vi "DDS Write Register.vi"(6 "channel number (1)":u8=1 min=1 max=4 step=1, 8 "error in (no error)":errorcluster, 9 "Write Data":u8[](array[numeric]), 10 "Register":T3, 11 "DDS ref in":T1={"NI USB-8451 device reference"="", "DIO port"=0, "Serial Clock Rate [kHz]"=1000}) -> (0 "error out":errorcluster, 3 "DDS ref out":T1={"NI USB-8451 device reference"="", "DIO port"=0, "Serial Clock Rate [kHz]"=1000})   [LabVIEW 2013]
doc: "Writes data to the specified register in the specified channel. The number of bytes written must equal the register size."
uses:
  AD9910 registers.ctl
  DDS_box_device_reference.ctl
  <vilib>/ni845x/ni845x.llb/ni845xControl.ctl
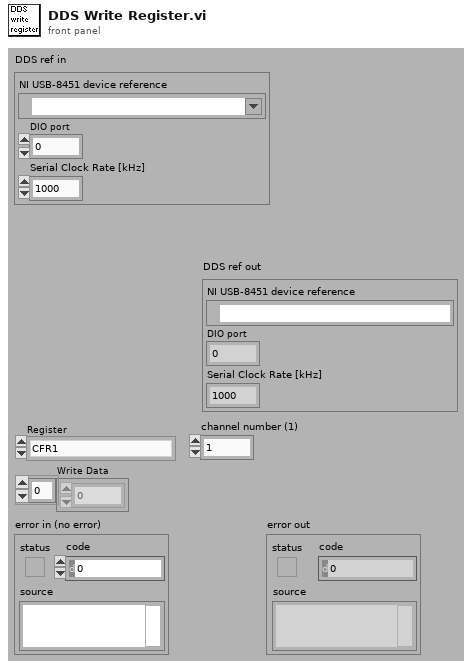
[diagram p1: front panel]
types:
  T1 = typedef "DDS_box_device_reference.ctl" = cluster{"NI USB-8451 device reference":T2, "DIO port":u8, "Serial Clock Rate [kHz]":u16}
  T2 = typedef "ni845xControl.ctl" = refnum<k21>
  T3 = typedef "AD9910 registers.ctl" = enum16{"CFR1", "CFR2", "CFR3", "Auxiliary DAC Control", "I/0 Update Rate", "Frequency Tuning Word", "Phase Offset Word", "Amplitude Scale Factor", "Multichip Sync", "Digital Ramp Limit", "Digital Ramp Step Size", "Digital Ramp Rate", "Single Tone Profile 0", "Single Tone Profile 1", "Single Tone Profile 2", "Single Tone Profile 3", "Single Tone Profile 4", "Single Tone Profile 5", "Single Tone Profile 6", "Single Tone Profile 7", "RAM Profile 0", "RAM Profile 1", "RAM Profile 2", "RAM Profile 3", "RAM Profile 4", "RAM Profile 5", "RAM Profile 6", "RAM Profile 7", "RAM"}
  T4 = typedef "ni845xSpiScriptControl.ctl" = refnum<k20>
  T5 = typedef "DDS CS pins.ctl" = enum8{"IO reset", "Ch. 4 CS", "Ch. 3 CS", "Ch. 2 CS", "Ch. 1 CS"}
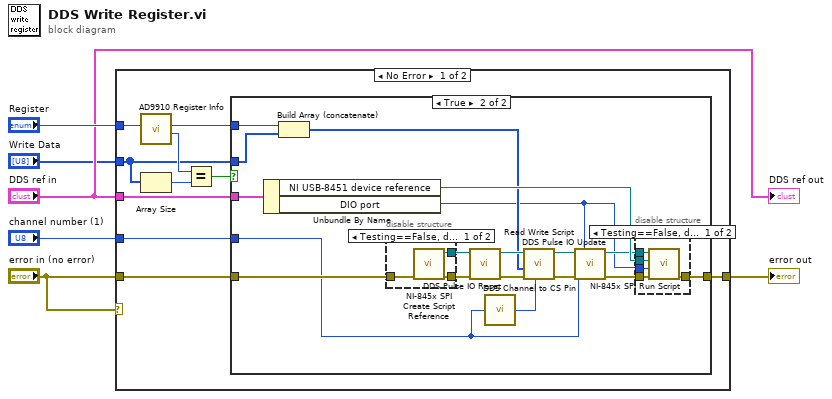
[diagram p0: block diagram]
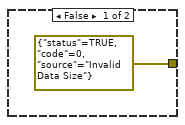
[diagram p2: hidden frame]
diagram:
  n1 = case shown="No Error" "error in (no error)" {
    tunnel: "error in (no error)" -> [w16 w46]
    tunnel: "DDS ref in" -> [w15 _]
    tunnel: "Register" -> [w14 _]
    tunnel: [w8 w46] -> w4
    tunnel: "Write Data" -> [w10 _]
    tunnel: "channel number (1)" -> [w7 _]
    frame No Error {
      n2 = call "AD9910 Register Info.vi"("Register"=w14) -> ("Number of Bytes"=w13:i32, "Address"=w9:u8)  [unwired: 9 in]
      n3 = Array Size(array=w10) -> (size(s)=w12:i32)
      n4 = Equal?(x=w13, y=w12) -> (x = y?=w11:bool)
      n5 = case shown="True" w11 {
        tunnel: w16 -> [_ w35]
        tunnel: w15 -> [_ w34]
        tunnel: w10 -> [_ w27]
        tunnel: w9 -> [_ w28]
        tunnel: [errorcluster {"status"=TRUE, "code"=0, "source"="Invalid Data Size"} ("error in (no error)") w25] -> w8
        tunnel: w7 -> [_ w20]
        frame False {
        }
        frame True {
          n6 = Unbundle By Name(w34) -> ("NI USB-8451 device reference"=w29:T2, "DIO port"=w18:u8)
          n7 = Build Array (concatenate)(w28, w27) -> (w26:u8[])
          n8 = disable-structure shown="Testing==False, default" {
            disable-tunnel: w35 -> [w44 w45]
            disable-tunnel: [w43 _] -> w33
            disable-tunnel: [w42 w45] -> w32
            frame condition #0 (active) {
              n9 = call <vilib>:"NI-845x SPI Create Script Reference.vi"("error in (no error)"=w44) -> ("error out"=w42:errorcluster, "spi script reference"=w43:T4)  [unwired: 9 in]
            }
            frame condition #1 {
            }
          }
          n10 = call "DDS Pulse IO Reset.vi"("error in (no error)"=w32, "spi script reference in"=w33) -> ("error out"=w31:errorcluster, "spi script reference out"=w30:T4)  [unwired: 8 in]
          n11 = call "DDS Channel to CS Pin.vi"("channel number (1)"=w20) -> ("CS pin"=w19:T5)
          n12 = call "Read Write Script.vi"("chip select (0)"=w19, "error in (no error)"=w31, "Write Data"=w26, "spi script reference in"=w30) -> ("error out"=w24:errorcluster, "spi script reference out"=w23:T4)  [unwired: 5 in, 1 out]
          n13 = call "DDS Pulse IO Update.vi"("port number (0)"=w18, "error in (no error)"=w24, "channel number (1)"=w20, "spi script reference in"=w23) -> ("error out"=w21:errorcluster, "spi script reference out"=w22:T4)  [unwired: 6 in]
          n14 = disable-structure shown="Testing==False, default" {
            disable-tunnel: w29 -> [w40 _]
            disable-tunnel: [w39 w41] -> w25
            disable-tunnel: w22 -> [w38 _]
            disable-tunnel: w21 -> [w37 w41]
            disable-tunnel: w18 -> [w36 _]
            frame condition #0 (active) {
              n15 = call <vilib>:"NI-845x SPI Run Script.vi"("error in (no error)"=w37, "port (0)"=w36, "device reference in"=w40, "spi script reference in"=w38) -> ("error out"=w39:errorcluster)  [unwired: 5 in, 2 out]
            }
            frame condition #1 {
            }
          }
        }
      }
    }
    frame Error {
    }
  }
  "error out" <- w4
  "DDS ref out" <- "DDS ref in"
